vi "Read CFG File.vi"(8 "error in (no error)":errorcluster, 10 "File path":path, 11 "Mag Lab Root in":refnum<class "Mag Lab Root.lvclass">) -> (0 "error out":errorcluster, 2 "Section":string, 3 "Mag Lab Root out":refnum<class "Mag Lab Root.lvclass">)   [LabVIEW 2015, in "Mag Lab Root.lvclass"]
uses:
  Mag Lab Root.lvclass
  Mag Lab Root.lvclass/Mag Lab Root.ctl
  Mag Lab Properties/Mag Lab Parameters.lvclass
  <vilib>/Utility/config.llb/NI_LVConfig.lvlib
  Mag Lab Error Handler/Mag Lab Error Handler.lvclass
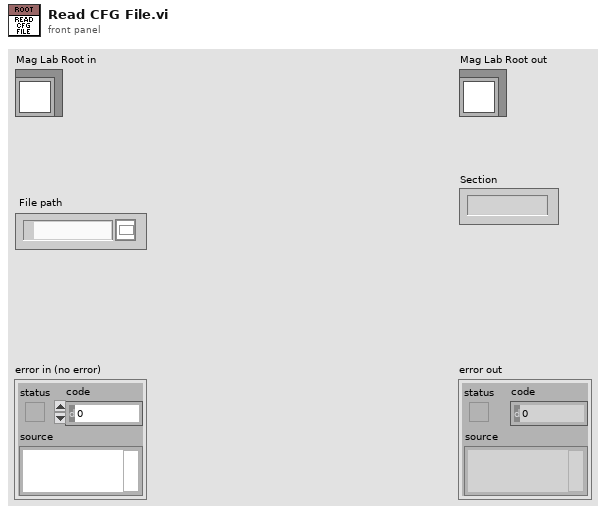
[diagram p1: front panel]
types:
  T1 = typedef "NI_LVConfig.lvlib/Config Data RefNum.ctl" = refnum<k1>
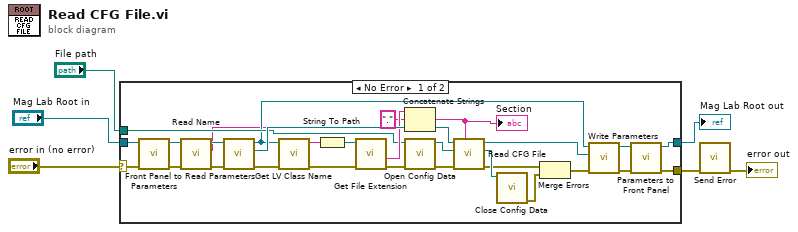
[diagram p0: block diagram]
diagram:
  n1 = case shown="No Error" "error in (no error)" {
    selector: "error in (no error)" -> [w25 w37]
    tunnel: [w20 w37] -> w5
    tunnel: [w22 w36] -> w3
    tunnel: "Mag Lab Root in" -> [w35 w36]
    tunnel: "File path" -> [w17 _]
    frame No Error {
      n2 = call-dynamic "Front Panel to Parameters.vi"("error in (no error)"=w25, "Mag Lab Root in"=w35) -> ("error out"=w32:errorcluster, "Mag Lab Root out"=w33:refnum<class "Mag Lab Root.lvclass">)  [unwired: 8 in]
      n3 = call "Read Name.vi"("error in (no error)"=w32, "Mag Lab Root in"=w33) -> ("error out"=w31:errorcluster, "Name"=w9:string, "Mag Lab Root out"=w34:refnum<class "Mag Lab Root.lvclass">)  [unwired: 7 in]
      n4 = call-dynamic "Read Parameters.vi"("error in (no error)"=w31, "Mag Lab Root in"=w34) -> ("error out"=w29:errorcluster, "Mag Lab Parameters.lvclass"=w30:refnum<class "Mag Lab Parameters.lvclass">, "Mag Lab Root out"=w14:refnum<class "Mag Lab Root.lvclass">)  [unwired: 7 in]
      n5 = call <vilib>:"Get LV Class Name.vi"("error in (no error)"=w29, "object"=w14) -> ("error out"=w24:errorcluster, "class name"=w13:string)  [unwired: 8 in]
      n6 = String To Path(string=w13) -> (path=w28:path)
      n7 = call <vilib>:"Get File Extension.vi"("error in (no error)"=w24, "file"=w28) -> ("error out"=w19:errorcluster, "filename without extension"=w27:string)  [unwired: 5 in, 3 out]
      n8 = Concatenate Strings(w27, "." ("string"), w9) -> (w7:string)
      "Section" <- w7
      n9 = call <vilib>:"Open Config Data.vi"("error in (no error)"=w19, "configuration file path"=w17) -> ("error out"=w15:errorcluster, "refnum"=w16:T1)  [unwired: 7 in, 1 out]
      n10 = call-dynamic "Read CFG File.vi"("Section"=w7, "error in (no error)"=w15, "File refnum"=w16, "Mag Lab Parameters in"=w30) -> ("error out"=w11:errorcluster, "File refnum out"=w18:T1, "Mag Lab Parameters out"=w26:refnum<class "Mag Lab Parameters.lvclass">)  [unwired: 5 in]
      n11 = call <vilib>:"Close Config Data.vi"("refnum"=w18) -> ("error out"=w12:errorcluster)  [unwired: 9 in, 1 out]
      n12 = Merge Errors(w11, w12) -> (w10:errorcluster)
      n13 = call-dynamic "Write Parameters.vi"("error in (no error)"=w10, "Mag Lab Parameters.lvclass"=w26, "Mag Lab Root in"=w14) -> ("error out"=w21:errorcluster, "Mag Lab Root out"=w23:refnum<class "Mag Lab Root.lvclass">)  [unwired: 7 in]
      n14 = call-dynamic "Parameters to Front Panel.vi"("error in (no error)"=w21, "Mag Lab Root in"=w23) -> ("error out"=w20:errorcluster, "Mag Lab Root out"=w22:refnum<class "Mag Lab Root.lvclass">)  [unwired: 8 in]
    }
    frame Error {
    }
  }
  "Mag Lab Root out" <- w3
  n15 = call "Send Error.vi"("error in (no error)"=w5) -> ("error out"=→"error out":errorcluster)  [unwired: 9 in, 1 out]
